vi "helper-io-set-tables.vi"(11 "IOnodes":T1[](array[typedef]) {"calibration"."Y" format="%#.3f"; "calibration"."X" format="%#.3f"; "ADDR" format="%04d"}) -> (0 "VL":T1[](array[typedef]) {"calibration"."Y" format="%#.3f"; "calibration"."X" format="%#.3f"; "ADDR" format="%04d"}, 1 "IO Map AI":T8[](array[typedef]) {"ADDR" format="%04d"}, 2 "IO Map DO":T7[](array[typedef]) {"ADDR" format="%04d"}, 3 "IO Map DI":T6[](array[typedef]) {"ADDR" format="%04d"})   [LabVIEW 2024]
uses:
  controls/type-io-map-ai.ctl
  controls/type.address.ctl
  controls/enum.io.mode.ctl
  controls/IONode.ctl
  controls/enum.io.type.ctl
  controls/typeXyPoint.ctl
  controls/type-io-map-do.ctl
  controls/type-io-map-di.ctl
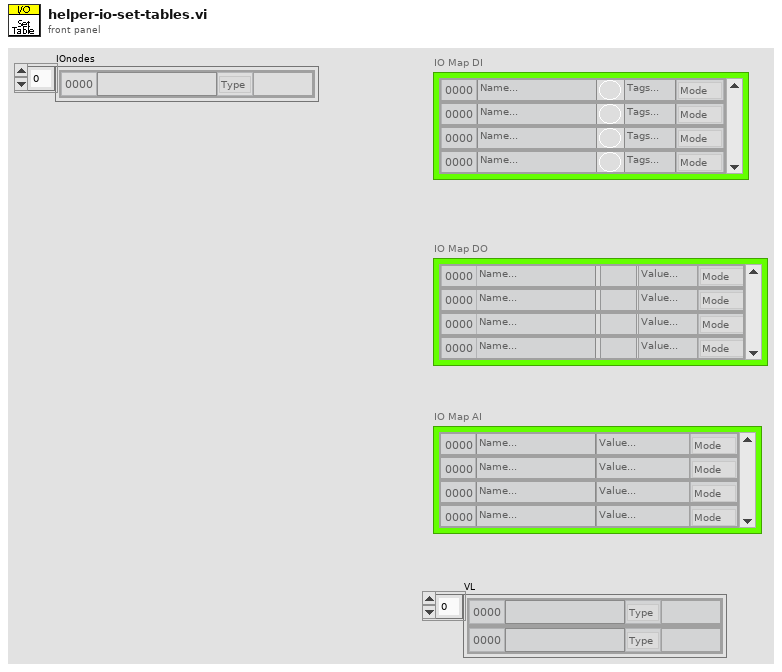
[diagram p1: front panel]
types:
  T1 = typedef "IONode.ctl" = cluster{"ADDR":T2, "Label":string, "Type":T3, "Mode":T4, "Value":string, "Tags":string, "calibration":T5[]}
  T2 = typedef "type.address.ctl" = u16
  T3 = typedef "enum.io.type.ctl" = enum16{"Type", "DI", "DO", "AI", "AO", "VL", "BUF"}
  T4 = typedef "enum.io.mode.ctl" = enum16{"Mode", "RIO", "SIM"}
  T5 = typedef "typeXyPoint.ctl" = cluster{"X":dbl, "Y":dbl}
  T6 = typedef "type-io-map-di.ctl" = cluster{"ADDR":T2, "Label":string, "Mode":T4, "State":bool, "Value":string}
  T7 = typedef "type-io-map-do.ctl" = cluster{"ADDR":T2, "Label":string, "Mode":T4, "Value":string, "State":bool}
  T8 = typedef "type-io-map-ai.ctl" = cluster{"ADDR":T2, "Label":string, "Mode":T4, "Value":string}
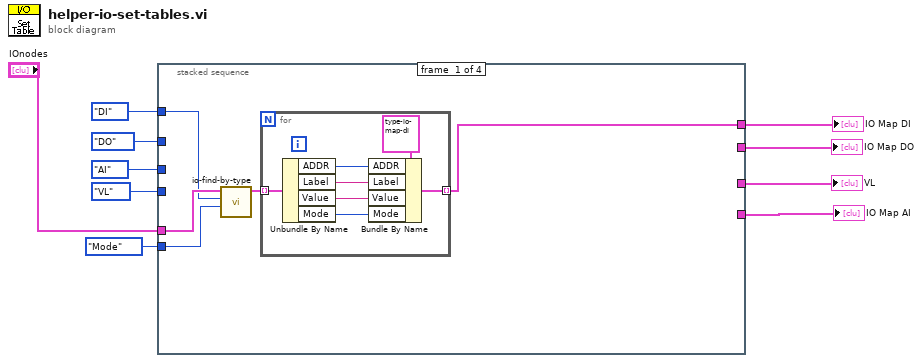
[diagram p0: block diagram]
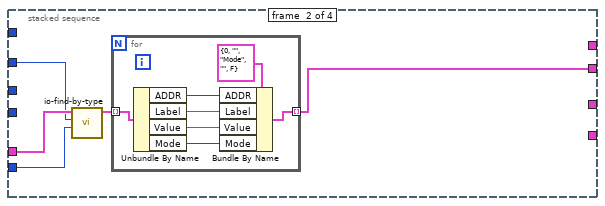
[diagram p2: hidden frame]
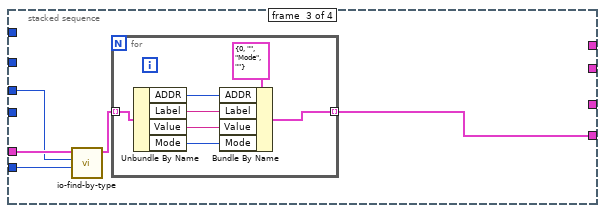
[diagram p3: hidden frame]
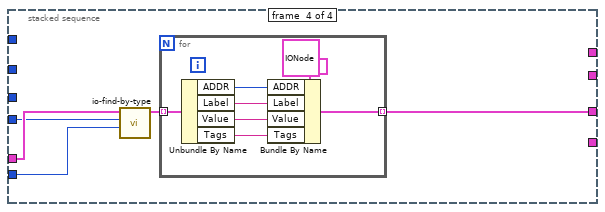
[diagram p4: hidden frame]
diagram:
  n1 = stacked-sequence {
    tunnel: "IOnodes" -> [w14 w26 w38 w50]
    tunnel: enum.io.mode."Mode" ("Mode(Any)") -> [w13 w25 w37 w48]
    tunnel: enum.io.type."VL" ("Type") -> [_ _ _ w49]
    tunnel: enum.io.type."DI" ("Type") -> [w12 _ _ _]
    tunnel: enum.io.type."AI" ("Type") -> [_ _ w36 _]
    tunnel: enum.io.type."DO" ("Type") -> [_ w24 _ _]
    tunnel: [w11 _ _ _] -> w7
    tunnel: [_ w23 _ _] -> w8
    tunnel: [_ _ w35 _] -> w10
    tunnel: [_ _ _ w47] -> w9
    frame #0 {
      n2 = call "io-find-by-type.vi"("Mode(Any)"=w13, "Type"=w12, "IOConfigs in"=w14) -> ("Search Results"=w15:T1[])  [unwired: 8 in]
      n3 = for {
        tunnel: w15 -> [w21] mode=indexing
        tunnel: [w22] -> w11 mode=indexing
        n4 = Unbundle By Name(w21) -> ("ADDR"=w20:T2, "Label"=w19:string, "Value"=w18:string, "Mode"=w16:T4)
        n5 = Bundle By Name(cluster=T6 {"ADDR"=0, "Label"="Name...", "Mode"=enum."Mode", "State"=FALSE, "Value"=""} ("IoConf in 3"), "ADDR"=w20, "Label"=w19, "Value"=w18, "Mode"=w16) -> (w22:T6)
      }
    }
    frame #1 {
      n6 = call "io-find-by-type.vi"("Mode(Any)"=w25, "Type"=w24, "IOConfigs in"=w26) -> ("Search Results"=w27:T1[])  [unwired: 8 in]
      n7 = for {
        tunnel: w27 -> [w33] mode=indexing
        tunnel: [w34] -> w23 mode=indexing
        n8 = Unbundle By Name(w33) -> ("ADDR"=w32:T2, "Label"=w31:string, "Value"=w30:string, "Mode"=w28:T4)
        n9 = Bundle By Name(cluster=T7 {"ADDR"=0, "Label"="", "Mode"=enum."Mode", "Value"="", "State"=FALSE} ("IO Map DO 2"), "ADDR"=w32, "Label"=w31, "Value"=w30, "Mode"=w28) -> (w34:T7)
      }
    }
    frame #2 {
      n10 = call "io-find-by-type.vi"("Mode(Any)"=w37, "Type"=w36, "IOConfigs in"=w38) -> ("Search Results"=w39:T1[])  [unwired: 8 in]
      n11 = for {
        tunnel: w39 -> [w45] mode=indexing
        tunnel: [w46] -> w35 mode=indexing
        n12 = Unbundle By Name(w45) -> ("ADDR"=w44:T2, "Label"=w43:string, "Value"=w42:string, "Mode"=w40:T4)
        n13 = Bundle By Name(cluster=T8 {"ADDR"=0, "Label"="", "Mode"=enum."Mode", "Value"=""} ("IoConf in 3"), "ADDR"=w44, "Label"=w43, "Value"=w42, "Mode"=w40) -> (w46:T8)
      }
    }
    frame #3 {
      n14 = call "io-find-by-type.vi"("Mode(Any)"=w48, "Type"=w49, "IOConfigs in"=w50) -> ("Search Results"=w51:T1[])  [unwired: 8 in]
      n15 = for {
        tunnel: w51 -> [w57] mode=indexing
        tunnel: [w58] -> w47 mode=indexing
        n16 = Unbundle By Name(w57) -> ("ADDR"=w56:T2, "Label"=w55:string, "Value"=w54:string, "Tags"=w53:string)
        n17 = Bundle By Name(cluster=T1 {"ADDR"=0, "Label"="Name", "Type"=enum."DI", "Mode"=enum."RIO", "Value"="Value", "Tags"="Tags", "calibration"=[]} ("IO Map VL"), "ADDR"=w56, "Label"=w55, "Value"=w54, "Tags"=w53) -> (w58:T1)
      }
    }
  }
  "IO Map AI" <- w10
  "VL" <- w9
  "IO Map DO" <- w8
  "IO Map DI" <- w7
